vi "ChapterTenFinalProject.vi"() -> ()   [LabVIEW 2010]
uses:
  <vilib>/Instr/_visa.llb/VISA Configure Serial Port (Instr).vi
  <vilib>/Utility/inputDevices.llb/closeJoystick.vi
  <vilib>/Utility/inputDevices.llb/joystickAcquire.vi
panel:
  in  "device index":i32=4
  in  "stop":bool
  out "Write Data":string
  in  "VISA resource name":refnum<visa-resource-name>
  out "error out":errorcluster
  in  "error in (no error)":errorcluster
  in  "Write":bool
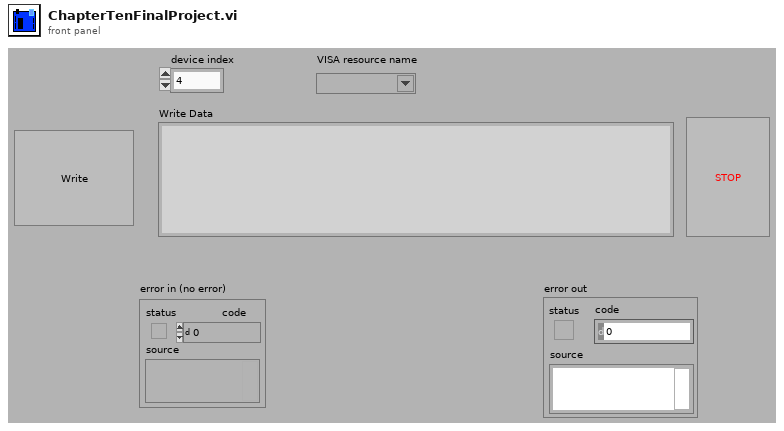
[diagram p1: front panel]
types:
  T1 = cluster{"X axis":i32, "Y axis":i32, "Z axis":i32, "X axis rotation":i32, "Y axis rotation":i32, "Z axis rotation":i32, "U axis":i32, "V axis":i32}
  T2 = cluster{"button 1":bool, "button 2":bool, "button 3":bool, "button 4":bool, "button 5":bool, "button 6":bool, "button 7":bool, "button 8":bool, "button 9":bool, "button 10":bool, "button 11":bool, "button 12":bool, "button 13":bool, "button 14":bool, "button 15":bool, "button 16":bool, "button 17":bool, "button 18":bool, "button 19":bool, "button 20":bool, "button 21":bool, "button 22":bool, "button 23":bool, "button 24":bool, "button 25":bool, "button 26":bool, "button 27":bool, "button 28":bool, "button 29":bool, "button 30":bool, "button 31":bool, "button 32":bool}
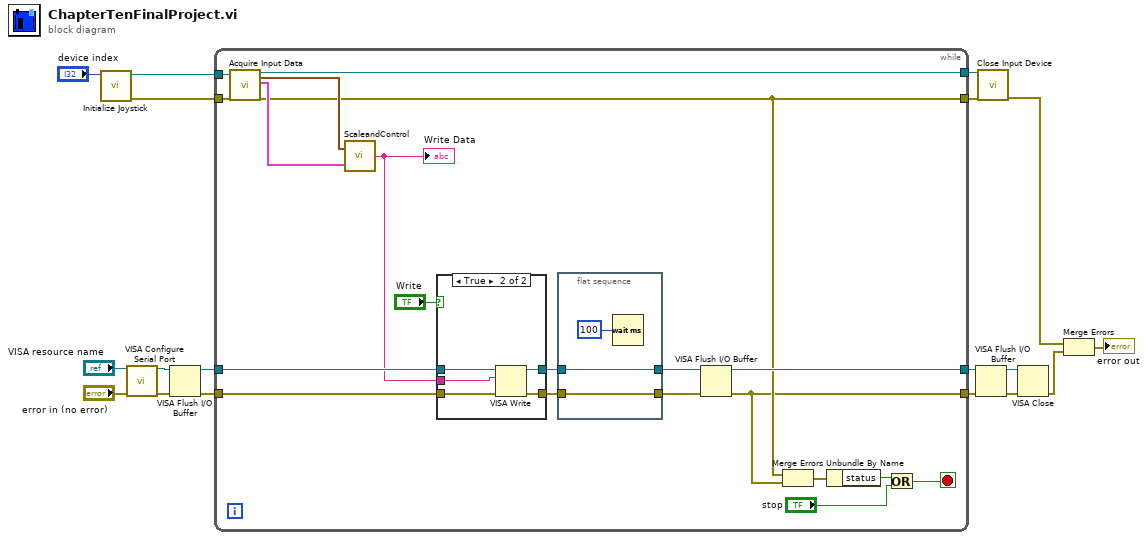
[diagram p0: block diagram]
diagram:
  n1 = call <vilib>:"Initialize Joystick.vi"("device index"="device index") -> ("error out"=w11:errorcluster, "device ID"=w12:refnum<k1>)  [unwired: 9 in]
  n2 = call-poly "VISA Configure Serial Port"("VISA resource name"="VISA resource name", "error in (no error)"="error in (no error)") -> ("VISA resource name out"=w13:refnum<visa-resource-name>, "error out"=w14:errorcluster)  [unwired: 12 in]
  n3 = VISA Flush I/O Buffer(VISA resource name=w13, error in (no error)=w14) -> (VISA resource name out=w8:refnum<visa-resource-name>, error out=w7:errorcluster)  [unwired: 1 in]
  n4 = while {
    tunnel: w12 -> [w37]
    tunnel: w11 -> [w36]
    tunnel: [w35] -> w10
    tunnel: [w20] -> w9
    tunnel: w8 -> [w28]
    tunnel: w7 -> [w27]
    tunnel: [w26] -> w6
    tunnel: [w19] -> w5
    stop <- w29 stop-if-true
    n5 = call-poly <vilib>:"Acquire Input Data.vi"("device ID"=w37, "error in (no error)"=w36) -> ("device ID"=w35:refnum<k1>, "axis info"=w38:T1, "button info"=w25:T2, "error out"=w20:errorcluster)  [unwired: 13 in, 1 out]
    n6 = call "ScaleandControl.vi"("button info"=w25, "axis info"=w38) -> ("String"=w24:string)
    "Write Data" <- w24
    n7 = case shown="True" "Write" {
      tunnel: [w43 w48] -> w33
      tunnel: [w42 w47] -> w34
      tunnel: w28 -> [w43 w46]
      tunnel: w27 -> [w42 w45]
      tunnel: w24 -> [_ w44]
      frame False {
      }
      frame True {
        n8 = VISA Write(VISA resource name=w46, write buffer=w44, error in (no error)=w45) -> (VISA resource name out=w48:refnum<visa-resource-name>, error out=w47:errorcluster)  [unwired: 1 out]
      }
    }
    n9 = flat-sequence {
      tunnel: w33 -> [w41]
      tunnel: [w41] -> w23
      tunnel: w34 -> [w40]
      tunnel: [w40] -> w22
      frame #0 {
        n10 = Wait (ms)(milliseconds to wait=u32 100) -> ()  [unwired: 1 out]
      }
    }
    n11 = VISA Flush I/O Buffer(VISA resource name=w23, error in (no error)=w22) -> (VISA resource name out=w26:refnum<visa-resource-name>, error out=w19:errorcluster)  [unwired: 1 in]
    n12 = Merge Errors(w20, w19) -> (w21:errorcluster)
    n13 = Unbundle By Name(w21) -> ("status"=w32:bool)
    n14 = Or(x=w32, y="stop") -> (x .or. y?=w29:bool)
  }
  n15 = VISA Flush I/O Buffer(VISA resource name=w6, error in (no error)=w5) -> (VISA resource name out=w15:refnum<visa-resource-name>, error out=w16:errorcluster)  [unwired: 1 in]
  n16 = call-poly <vilib>:"Close Input Device.vi"("error in (no error)"=w9, "device ID"=w10) -> ("error out"=w1:errorcluster)  [unwired: 8 in]
  n17 = VISA Close(VISA resource name=w15, error in (no error)=w16) -> (error out=w3:errorcluster)
  n18 = Merge Errors(w1, w3) -> (→"error out":errorcluster)
